vi "test_config_file_generator.vi"() -> ()   [LabVIEW 2019]
uses:
  RT/RT Controls/Main Box Config.ctl
  <vilib>/Utility/config.llb/Config Data RefNum.ctl
  <vilib>/Utility/config.llb/Write Key (I32).vi
  <vilib>/Utility/config.llb/Write Key (Double).vi
  <vilib>/Utility/config.llb/Write Key (Boolean).vi
  <vilib>/Utility/config.llb/Write Key (U32).vi
  <vilib>/Utility/config.llb/Read Key (I32).vi
  <vilib>/Utility/config.llb/Read Key (Double).vi
  <vilib>/Utility/config.llb/Read Key (Boolean).vi
  <vilib>/Utility/config.llb/NI_LVConfig.lvlib
panel:
  out "out":T2 {"MainBoxConfig"."Tol" format="%.2f"; "MainBoxConfig"."EncRefDeg" format="%.2f"; "MainBoxConfig"."HomePos" format="%.2f"; "MainBoxConfig"."HSThres" format="%.2f"; "MainBoxConfig"."Coast" format="%.2f"}
  in  "AzEncNoError":u16=1025
  out "error out":errorcluster
  out "key names":string[](array[string])
  out "section exists?":bool
  out "file refnum":T3
  in  "MainHostTO":u16=60
  in  "MainHostPort":u16=17310
  in  "TopUDPPort":u16=17308
  in  "config path":path=path "C:/Users/norman/Documents/test/soar_dome/test/config.ini"
  in  "MainBoxConfig":T1={"WatchdogTim"=600, "DirRevDel"=4, "Coast"=0.5, "HSThres"=5.0, "EncCounts360"=4018143232, "HomePos"=0.0, "EncRefDeg"=0.0, "EncRefCounts"=79895940197, "Tol"=1.0, "CloudEn"=FALSE, "AutoShutEn"=FALSE, "RainTim"=5, "AZTimeout"=120, "AZEncPol"=enum."Positive"} caption="value" {"Tol" format="%.2f"; "EncRefDeg" format="%.2f"; "HomePos" format="%.2f"; "HSThres" format="%.2f"; "Coast" format="%.2f"}
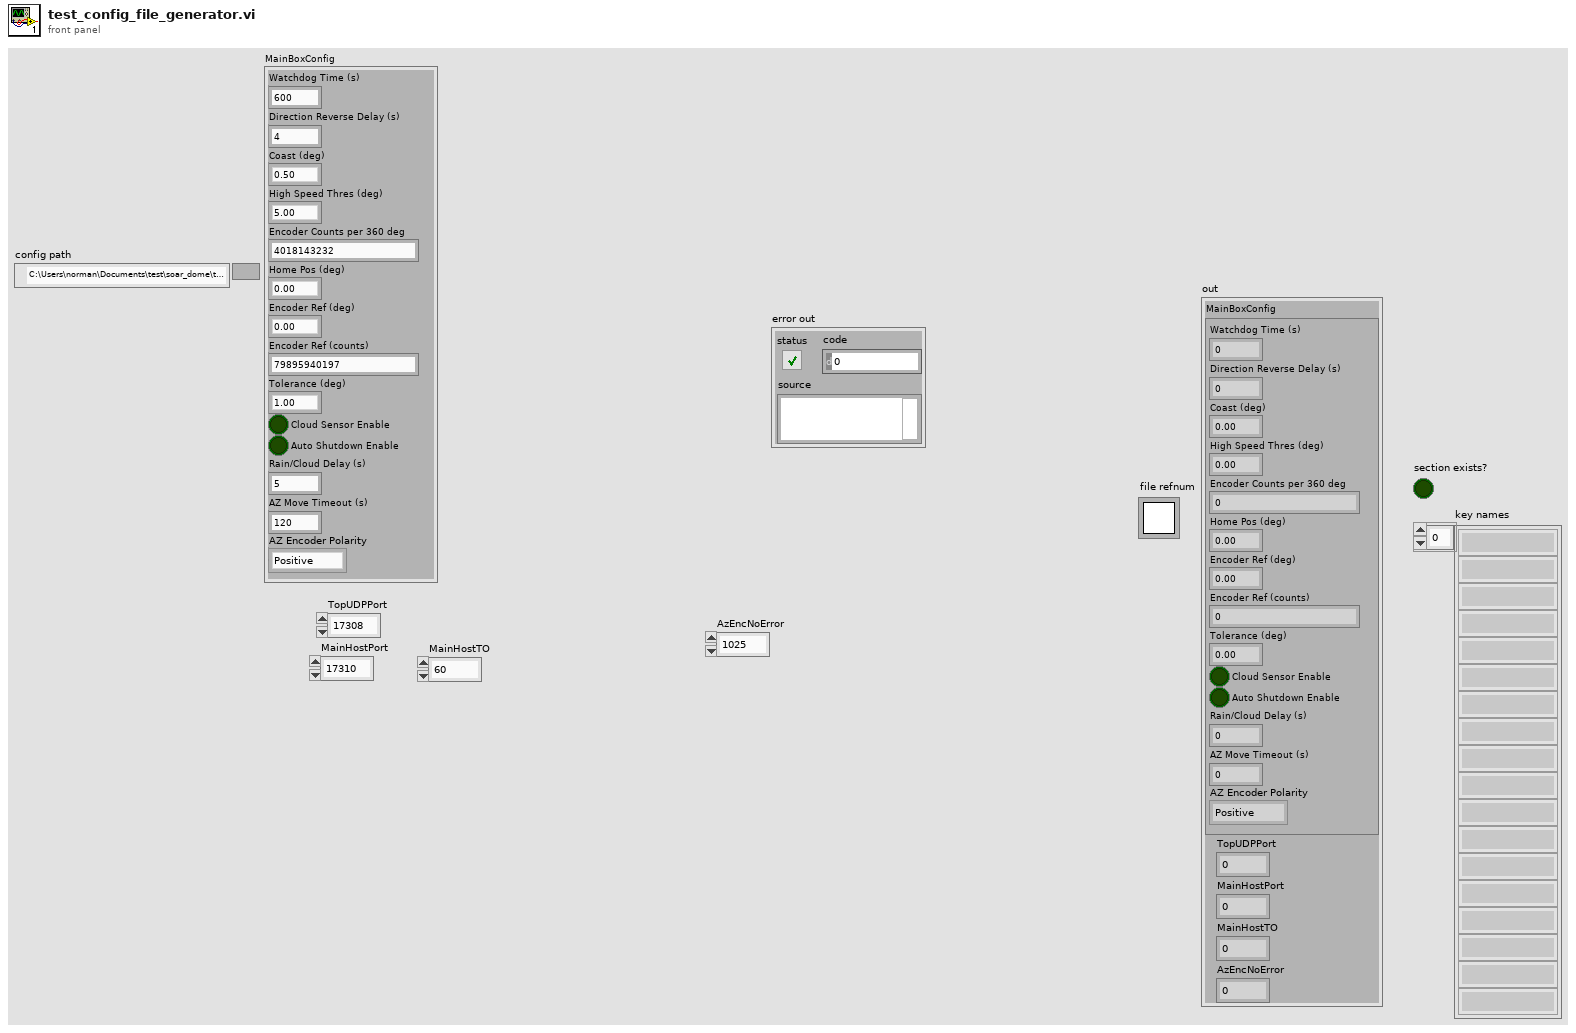
[diagram p1: front panel]
types:
  T1 = typedef "Main Box Config.ctl" = cluster{"WatchdogTim":i32, "DirRevDel":i32, "Coast":dbl, "HSThres":dbl, "EncCounts360":u64, "HomePos":dbl, "EncRefDeg":dbl, "EncRefCounts":u64, "Tol":dbl, "CloudEn":bool, "AutoShutEn":bool, "RainTim":i32, "AZTimeout":i32, "AZEncPol":enum16{"Positive", "Negative"}}
  T2 = cluster{"MainBoxConfig":T1, "TopUDPPort":u16, "MainHostPort":u16, "MainHostTO":u16, "AzEncNoError":u16}
  T3 = typedef "NI_LVConfig.lvlib/Config Data RefNum.ctl" = refnum<k1>
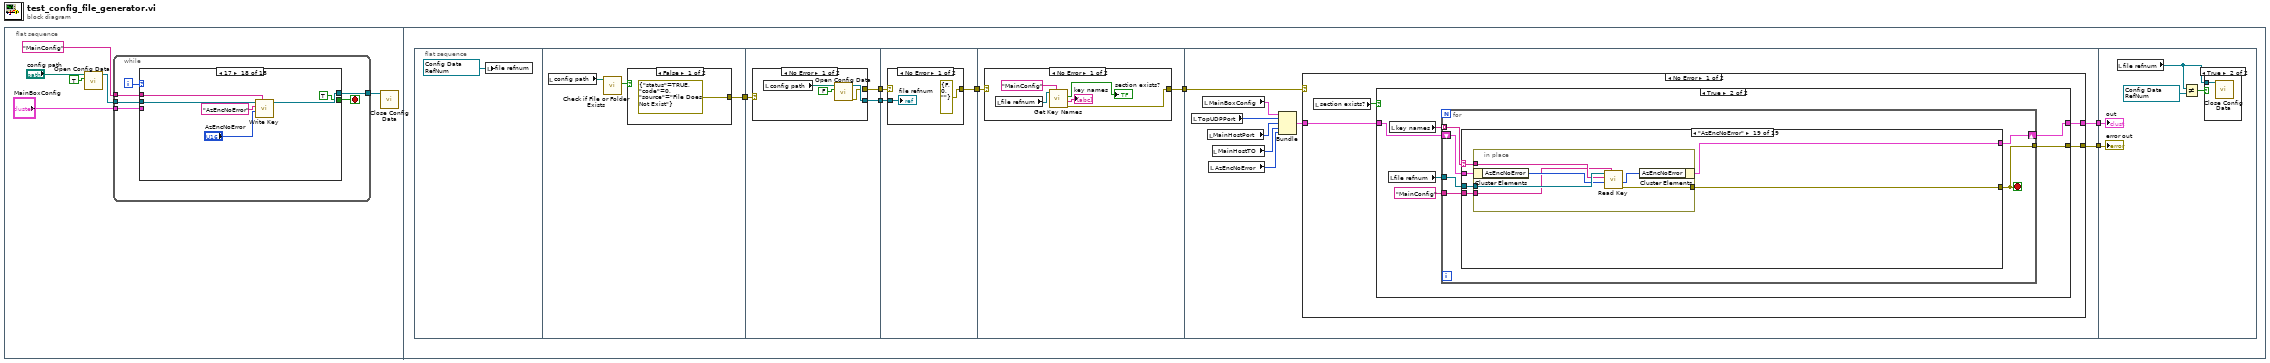
[diagram p0: block diagram]
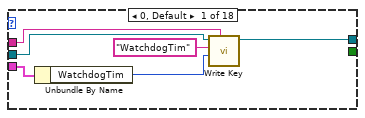
[diagram p2: hidden frame]
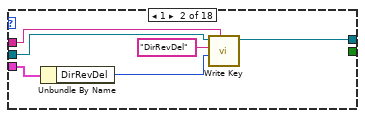
[diagram p3: hidden frame]
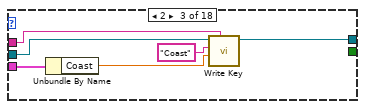
[diagram p4: hidden frame]
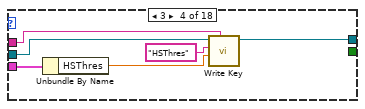
[diagram p5: hidden frame]
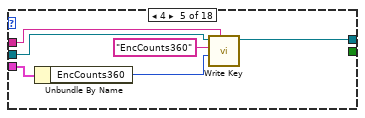
[diagram p6: hidden frame]
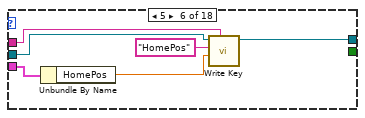
[diagram p7: hidden frame]
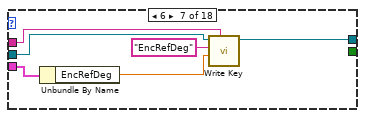
[diagram p8: hidden frame]
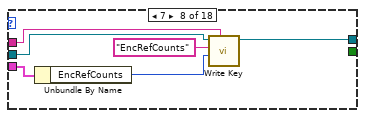
[diagram p9: hidden frame]
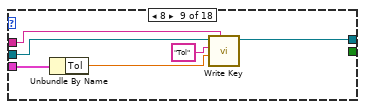
[diagram p10: hidden frame]
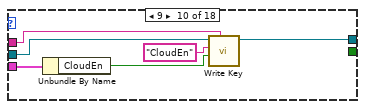
[diagram p11: hidden frame]
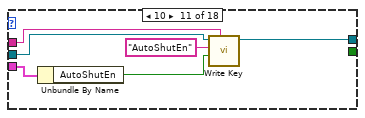
[diagram p12: hidden frame]
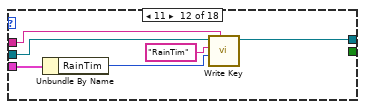
[diagram p13: hidden frame]
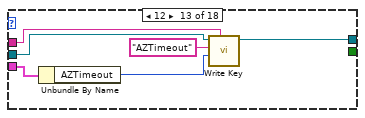
[diagram p14: hidden frame]
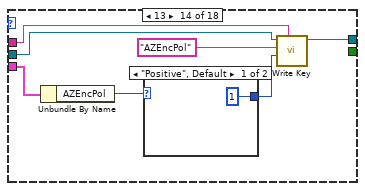
[diagram p15: hidden frame]
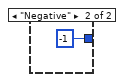
[diagram p16: hidden frame]
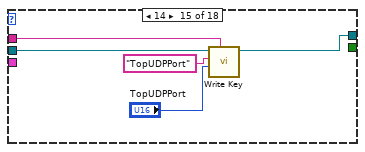
[diagram p17: hidden frame]
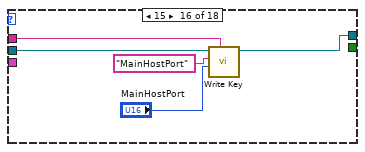
[diagram p18: hidden frame]
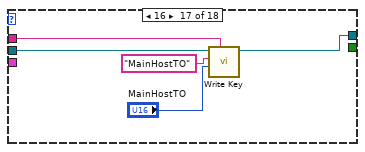
[diagram p19: hidden frame]
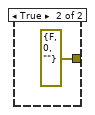
[diagram p20: hidden frame]
diagram:
  n1 = flat-sequence {
    frame #0 {
      n2 = call <vilib>:"Open Config Data.vi"("create file if necessary (T)"=TRUE, "configuration file path"="config path") -> ("refnum"=w4:T3)  [unwired: 7 in, 2 out]
      n3 = while {
        tunnel: w4 -> [w10]
        tunnel: "MainConfig" ("section") -> [w11]
        tunnel: [w9] -> w1
        tunnel: "MainBoxConfig" -> [w8]
        i -> [w12]
        stop <- w7 stop-if-true
        n4 = case shown="17" w12 {
          tunnel: w11 -> [w18 w24 w30 w36 w42 w48 w54 w60 w66 w72 w78 w84 w90 w97 w103 w108 w113 w119]
          tunnel: w10 -> [w17 w23 w29 w35 w41 w47 w53 w59 w65 w71 w77 w83 w89 w96 w104 w109 w114 w120]
          tunnel: [w16 w22 w28 w34 w40 w46 w52 w58 w64 w70 w76 w82 w88 w95 w100 w106 w111 w117] -> w9
          tunnel: w8 -> [w14 w20 w26 w32 w38 w44 w50 w56 w62 w68 w74 w80 w86 w93 _ _ _ _]
          tunnel: [_ _ _ _ _ _ _ _ _ _ _ _ _ _ _ _ _ TRUE] -> w7
          frame 0, Default {
            n5 = Unbundle By Name(w14) -> ("WatchdogTim"=w13:i32)
            n6 = call-poly <vilib>:"Write Key.vi"("section"=w18, "value"=w13, "key"="WatchdogTim", "refnum"=w17) -> ("refnum out"=w16:T3)  [unwired: 5 in, 2 out]
          }
          frame 1 {
            n7 = Unbundle By Name(w20) -> ("DirRevDel"=w19:i32)
            n8 = call-poly <vilib>:"Write Key.vi"("section"=w24, "value"=w19, "key"="DirRevDel", "refnum"=w23) -> ("refnum out"=w22:T3)  [unwired: 5 in, 2 out]
          }
          frame 2 {
            n9 = Unbundle By Name(w26) -> ("Coast"=w25:dbl)
            n10 = call-poly <vilib>:"Write Key.vi"("section"=w30, "value"=w25, "key"="Coast", "refnum"=w29) -> ("refnum out"=w28:T3)  [unwired: 5 in, 2 out]
          }
          frame 3 {
            n11 = Unbundle By Name(w32) -> ("HSThres"=w31:dbl)
            n12 = call-poly <vilib>:"Write Key.vi"("section"=w36, "value"=w31, "key"="HSThres", "refnum"=w35) -> ("refnum out"=w34:T3)  [unwired: 5 in, 2 out]
          }
          frame 4 {
            n13 = Unbundle By Name(w38) -> ("EncCounts360"=w37:u64)
            n14 = call-poly <vilib>:"Write Key.vi"("section"=w42, "value"=w37, "key"="EncCounts360", "refnum"=w41) -> ("refnum out"=w40:T3)  [unwired: 5 in, 2 out]
          }
          frame 5 {
            n15 = Unbundle By Name(w44) -> ("HomePos"=w43:dbl)
            n16 = call-poly <vilib>:"Write Key.vi"("section"=w48, "value"=w43, "key"="HomePos", "refnum"=w47) -> ("refnum out"=w46:T3)  [unwired: 5 in, 2 out]
          }
          frame 6 {
            n17 = Unbundle By Name(w50) -> ("EncRefDeg"=w49:dbl)
            n18 = call-poly <vilib>:"Write Key.vi"("section"=w54, "value"=w49, "key"="EncRefDeg", "refnum"=w53) -> ("refnum out"=w52:T3)  [unwired: 5 in, 2 out]
          }
          frame 7 {
            n19 = Unbundle By Name(w56) -> ("EncRefCounts"=w55:u64)
            n20 = call-poly <vilib>:"Write Key.vi"("section"=w60, "value"=w55, "key"="EncRefCounts", "refnum"=w59) -> ("refnum out"=w58:T3)  [unwired: 5 in, 2 out]
          }
          frame 8 {
            n21 = Unbundle By Name(w62) -> ("Tol"=w61:dbl)
            n22 = call-poly <vilib>:"Write Key.vi"("section"=w66, "value"=w61, "key"="Tol", "refnum"=w65) -> ("refnum out"=w64:T3)  [unwired: 5 in, 2 out]
          }
          frame 9 {
            n23 = Unbundle By Name(w68) -> ("CloudEn"=w67:bool)
            n24 = call-poly <vilib>:"Write Key.vi"("section"=w72, "value"=w67, "key"="CloudEn", "refnum"=w71) -> ("refnum out"=w70:T3)  [unwired: 5 in, 2 out]
          }
          frame 10 {
            n25 = Unbundle By Name(w74) -> ("AutoShutEn"=w73:bool)
            n26 = call-poly <vilib>:"Write Key.vi"("section"=w78, "value"=w73, "key"="AutoShutEn", "refnum"=w77) -> ("refnum out"=w76:T3)  [unwired: 5 in, 2 out]
          }
          frame 11 {
            n27 = Unbundle By Name(w80) -> ("RainTim"=w79:i32)
            n28 = call-poly <vilib>:"Write Key.vi"("section"=w84, "value"=w79, "key"="RainTim", "refnum"=w83) -> ("refnum out"=w82:T3)  [unwired: 5 in, 2 out]
          }
          frame 12 {
            n29 = Unbundle By Name(w86) -> ("AZTimeout"=w85:i32)
            n30 = call-poly <vilib>:"Write Key.vi"("section"=w90, "value"=w85, "key"="AZTimeout", "refnum"=w89) -> ("refnum out"=w88:T3)  [unwired: 5 in, 2 out]
          }
          frame 13 {
            n31 = Unbundle By Name(w93) -> ("AZEncPol"=w92:enum16{"Positive", "Negative"})
            n32 = case shown="\"Positive\", Default" w92 {
              tunnel: [1 -1] -> w91
              frame "Positive", Default {
              }
              frame "Negative" {
              }
            }
            n33 = call-poly <vilib>:"Write Key.vi"("section"=w97, "value"=w91, "key"="AZEncPol", "refnum"=w96) -> ("refnum out"=w95:T3)  [unwired: 5 in, 2 out]
          }
          frame 14 {
            n34 = call-poly <vilib>:"Write Key.vi"("section"=w103, "value"="TopUDPPort", "key"="TopUDPPort", "refnum"=w104) -> ("refnum out"=w100:T3)  [unwired: 5 in, 2 out]
          }
          frame 15 {
            n35 = call-poly <vilib>:"Write Key.vi"("section"=w108, "value"="MainHostPort", "key"="MainHostPort", "refnum"=w109) -> ("refnum out"=w106:T3)  [unwired: 5 in, 2 out]
          }
          frame 16 {
            n36 = call-poly <vilib>:"Write Key.vi"("section"=w113, "value"="MainHostTO", "key"="MainHostTO", "refnum"=w114) -> ("refnum out"=w111:T3)  [unwired: 5 in, 2 out]
          }
          frame 17 {
            n37 = call-poly <vilib>:"Write Key.vi"("section"=w119, "value"="AzEncNoError", "key"="AzEncNoError", "refnum"=w120) -> ("refnum out"=w117:T3)  [unwired: 5 in, 2 out]
          }
        }
      }
      n38 = call <vilib>:"Close Config Data.vi"("refnum"=w1) -> ()  [unwired: 9 in, 2 out]
    }
    frame #1 {
      n39 = flat-sequence {
        tunnel: [w129] -> w127
        tunnel: w127 -> [w136]
        tunnel: [w135] -> w126
        tunnel: [w134] -> w125
        tunnel: w126 -> [w144]
        tunnel: w125 -> [w145]
        tunnel: [w143] -> w124
        tunnel: w124 -> [w150]
        tunnel: [w149] -> w123
        tunnel: w123 -> [w160]
        tunnel: [w159] -> w122
        tunnel: [w158] -> w121
        tunnel: w122 -> [w414]
        tunnel: w121 -> [w410]
        frame #0 {
          w128 = T3 refnum items=["config data"] ("file refnum")
          n40 = local write "file refnum"(w128) -> ()
        }
        frame #1 {
          n41 = local read "config path"() -> (w130:path)
          n42 = call <vilib>:"Check if File or Folder Exists.vi"("path"=w130) -> ("file or folder exists?"=w131:bool)  [unwired: 8 in, 2 out]
          n43 = case shown="False" w131 {
            tunnel: [errorcluster {"status"=TRUE, "code"=0, "source"="File Does Not Exist"} ("error constant") errorcluster {"status"=FALSE, "code"=0, "source"=""} ("error constant")] -> w129
            frame False {
            }
            frame True {
            }
          }
        }
        frame #2 {
          n44 = case shown="No Error" w136 {
            selector: w136 -> [_ w141]
            tunnel: [w139 w142] -> w135
            tunnel: [w138 w141] -> w134
            frame No Error {
              n45 = local read "config path"() -> (w140:path)
              n46 = call <vilib>:"Open Config Data.vi"("create file if necessary (T)"=FALSE, "configuration file path"=w140) -> ("error out"=w138:errorcluster, "refnum"=w139:T3)  [unwired: 7 in, 1 out]
            }
            frame Error {
              w142 = T3 refnum items=["config data"] ("refnum")
            }
          }
        }
        frame #3 {
          n47 = case shown="No Error" w145 {
            selector: w145 -> [_ w148]
            tunnel: w144 -> [w147 _]
            tunnel: [errorcluster {"status"=FALSE, "code"=0, "source"=""} ("error IO") w148] -> w143
            frame No Error {
              "file refnum" <- w147
            }
            frame Error {
            }
          }
        }
        frame #4 {
          n48 = case shown="No Error" w150 {
            selector: w150 -> [_ w156]
            tunnel: [w153 w156] -> w149
            frame No Error {
              n49 = local read "file refnum"() -> (w155:T3)
              n50 = call <vilib>:"Get Key Names.vi"("section"="MainConfig", "refnum"=w155) -> ("error out"=w153:errorcluster, "key names"=→"key names":string[], "section exists?"=→"section exists?":bool)  [unwired: 6 in, 1 out]
            }
            frame Error {
            }
          }
        }
        frame #5 {
          n51 = local read "TopUDPPort"() -> (w163:u16)
          n52 = local read "MainBoxConfig"() -> (w164:T1)
          n53 = local read "MainHostPort"() -> (w162:u16)
          n54 = local read "AzEncNoError"() -> (w157:u16)
          n55 = local read "MainHostTO"() -> (w161:u16)
          n56 = Bundle("MainBoxConfig"=w164, "TopUDPPort"=w163, "MainHostPort"=w162, "MainHostTO"=w161, "AzEncNoError"=w157) -> (w165:T2)  [unwired: 1 in]
          n57 = case shown="No Error" w160 {
            selector: w160 -> [_ w408]
            tunnel: [w169 w409] -> w158
            tunnel: w165 -> [w168 w409]
            tunnel: [w166 w408] -> w159
            frame No Error {
              n58 = local read "section exists?"() -> (w167:bool)
              n59 = case shown="True" w167 {
                tunnel: w168 -> [w171 w177]
                tunnel: [w171 w176] -> w169
                tunnel: [errorcluster {"status"=FALSE, "code"=0, "source"=""} ("error out") w175] -> w166
                frame False {
                }
                frame True {
                  n60 = local read "file refnum"() -> (w172:T3)
                  n61 = local read "key names"() -> (w174:string[])
                  n62 = for {
                    tunnel: w174 -> [w183] mode=indexing
                    tunnel: w172 -> [w182]
                    shift-right: [w180] -> w176
                    shift-left: w177 -> [w181]
                    tunnel: "MainConfig" ("section") -> [w179]
                    tunnel: [w178] -> w175
                    stop <- w178 stop-if-true
                    n63 = case shown="\"AzEncNoError\"" w183 {
                      selector: w183 -> [_ w188 w200 w212 w224 w235 w247 w259 w271 w283 w295 w307 w319 w331 w343 w361 w373 w385 w397]
                      tunnel: w182 -> [_ w189 w201 w213 w225 w237 w249 w261 w273 w285 w297 w309 w321 w333 w345 w362 w374 w386 w398]
                      tunnel: w181 -> [w185 w191 w203 w215 w227 w239 w251 w263 w275 w287 w299 w311 w323 w335 w347 w365 w377 w389 w401]
                      tunnel: [w185 w190 w202 w214 w226 w238 w250 w262 w274 w286 w298 w310 w322 w334 w346 w364 w376 w388 w400] -> w180
                      tunnel: w179 -> [_ w187 w199 w211 w223 w236 w248 w260 w272 w284 w296 w308 w320 w332 w344 w363 w375 w387 w399]
                      tunnel: [errorcluster {"status"=FALSE, "code"=0, "source"=""} ("error out") w186 w198 w210 w222 w234 w246 w258 w270 w282 w294 w306 w318 w330 w342 w360 w372 w384 w396] -> w178
                      frame "False", Default {
                      }
                      frame "WatchdogTim" {
                        n64 = in-place {
                          in-place-border: w189 -> [w197]
                          in-place-border: w188 -> [w194]
                          in-place-border: w187 -> [w193]
                          in-place-border: [w192] -> w186
                          n65 = in-place-cluster #1(w191) -> ("MainBoxConfig.WatchdogTim"=w196:i32)
                          n66 = call-poly <vilib>:"Read Key.vi"("section"=w193, "default value"=w196, "key"=w194, "refnum"=w197) -> ("error out"=w192:errorcluster, "value"=w195:i32)  [unwired: 4 in, 2 out]
                          n67 = in-place-cluster #1("MainBoxConfig.WatchdogTim"=w195) -> (w190:T2)
                        }
                      }
                      frame "DirRevDel" {
                        n68 = in-place {
                          in-place-border: w201 -> [w209]
                          in-place-border: w200 -> [w206]
                          in-place-border: w199 -> [w205]
                          in-place-border: [w204] -> w198
                          n69 = in-place-cluster #2(w203) -> ("MainBoxConfig.DirRevDel"=w208:i32)
                          n70 = call-poly <vilib>:"Read Key.vi"("section"=w205, "default value"=w208, "key"=w206, "refnum"=w209) -> ("error out"=w204:errorcluster, "value"=w207:i32)  [unwired: 4 in, 2 out]
                          n71 = in-place-cluster #2("MainBoxConfig.DirRevDel"=w207) -> (w202:T2)
                        }
                      }
                      frame "Coast" {
                        n72 = in-place {
                          in-place-border: w213 -> [w221]
                          in-place-border: w212 -> [w218]
                          in-place-border: w211 -> [w217]
                          in-place-border: [w216] -> w210
                          n73 = in-place-cluster #3(w215) -> ("MainBoxConfig.Coast"=w220:dbl)
                          n74 = call-poly <vilib>:"Read Key.vi"("section"=w217, "default value"=w220, "key"=w218, "refnum"=w221) -> ("error out"=w216:errorcluster, "value"=w219:dbl)  [unwired: 4 in, 2 out]
                          n75 = in-place-cluster #3("MainBoxConfig.Coast"=w219) -> (w214:T2)
                        }
                      }
                      frame "HSThres" {
                        n76 = in-place {
                          in-place-border: w225 -> [w233]
                          in-place-border: w224 -> [w230]
                          in-place-border: w223 -> [w229]
                          in-place-border: [w228] -> w222
                          n77 = in-place-cluster #4(w227) -> ("MainBoxConfig.HSThres"=w232:dbl)
                          n78 = call-poly <vilib>:"Read Key.vi"("section"=w229, "default value"=w232, "key"=w230, "refnum"=w233) -> ("error out"=w228:errorcluster, "value"=w231:dbl)  [unwired: 4 in, 2 out]
                          n79 = in-place-cluster #4("MainBoxConfig.HSThres"=w231) -> (w226:T2)
                        }
                      }
                      frame "EncCounts360" {
                        n80 = in-place {
                          in-place-border: w237 -> [w245]
                          in-place-border: w236 -> [w242]
                          in-place-border: w235 -> [w241]
                          in-place-border: [w240] -> w234
                          n81 = in-place-cluster #5(w239) -> ("MainBoxConfig.EncCounts360"=w244:u64)
                          n82 = call-poly <vilib>:"Read Key.vi"("section"=w242, "default value"=w244, "key"=w241, "refnum"=w245) -> ("error out"=w240:errorcluster, "value"=w243:dbl)  [unwired: 4 in, 2 out]
                          n83 = in-place-cluster #5("MainBoxConfig.EncCounts360"=w243) -> (w238:T2)
                        }
                      }
                      frame "HomePos" {
                        n84 = in-place {
                          in-place-border: w249 -> [w257]
                          in-place-border: w248 -> [w254]
                          in-place-border: w247 -> [w253]
                          in-place-border: [w252] -> w246
                          n85 = in-place-cluster #6(w251) -> ("MainBoxConfig.HomePos"=w256:dbl)
                          n86 = call-poly <vilib>:"Read Key.vi"("section"=w254, "default value"=w256, "key"=w253, "refnum"=w257) -> ("error out"=w252:errorcluster, "value"=w255:dbl)  [unwired: 4 in, 2 out]
                          n87 = in-place-cluster #6("MainBoxConfig.HomePos"=w255) -> (w250:T2)
                        }
                      }
                      frame "EncRefDeg" {
                        n88 = in-place {
                          in-place-border: w261 -> [w269]
                          in-place-border: w260 -> [w266]
                          in-place-border: w259 -> [w265]
                          in-place-border: [w264] -> w258
                          n89 = in-place-cluster #7(w263) -> ("MainBoxConfig.EncRefDeg"=w268:dbl)
                          n90 = call-poly <vilib>:"Read Key.vi"("section"=w266, "default value"=w268, "key"=w265, "refnum"=w269) -> ("error out"=w264:errorcluster, "value"=w267:dbl)  [unwired: 4 in, 2 out]
                          n91 = in-place-cluster #7("MainBoxConfig.EncRefDeg"=w267) -> (w262:T2)
                        }
                      }
                      frame "EncRefCounts" {
                        n92 = in-place {
                          in-place-border: w273 -> [w281]
                          in-place-border: w272 -> [w278]
                          in-place-border: w271 -> [w277]
                          in-place-border: [w276] -> w270
                          n93 = in-place-cluster #8(w275) -> ("MainBoxConfig.EncRefCounts"=w280:u64)
                          n94 = call-poly <vilib>:"Read Key.vi"("section"=w278, "default value"=w280, "key"=w277, "refnum"=w281) -> ("error out"=w276:errorcluster, "value"=w279:dbl)  [unwired: 4 in, 2 out]
                          n95 = in-place-cluster #8("MainBoxConfig.EncRefCounts"=w279) -> (w274:T2)
                        }
                      }
                      frame "Tol" {
                        n96 = in-place {
                          in-place-border: w285 -> [w293]
                          in-place-border: w284 -> [w290]
                          in-place-border: w283 -> [w289]
                          in-place-border: [w288] -> w282
                          n97 = in-place-cluster #9(w287) -> ("MainBoxConfig.Tol"=w292:dbl)
                          n98 = call-poly <vilib>:"Read Key.vi"("section"=w290, "default value"=w292, "key"=w289, "refnum"=w293) -> ("error out"=w288:errorcluster, "value"=w291:dbl)  [unwired: 4 in, 2 out]
                          n99 = in-place-cluster #9("MainBoxConfig.Tol"=w291) -> (w286:T2)
                        }
                      }
                      frame "CloudEn" {
                        n100 = in-place {
                          in-place-border: w297 -> [w305]
                          in-place-border: w296 -> [w302]
                          in-place-border: w295 -> [w301]
                          in-place-border: [w300] -> w294
                          n101 = in-place-cluster #10(w299) -> ("MainBoxConfig.CloudEn"=w304:bool)
                          n102 = call-poly <vilib>:"Read Key.vi"("section"=w302, "default value"=w304, "key"=w301, "refnum"=w305) -> ("error out"=w300:errorcluster, "value"=w303:bool)  [unwired: 4 in, 2 out]
                          n103 = in-place-cluster #10("MainBoxConfig.CloudEn"=w303) -> (w298:T2)
                        }
                      }
                      frame "AutoShutEn" {
                        n104 = in-place {
                          in-place-border: w309 -> [w317]
                          in-place-border: w308 -> [w314]
                          in-place-border: w307 -> [w313]
                          in-place-border: [w312] -> w306
                          n105 = in-place-cluster #11(w311) -> ("MainBoxConfig.AutoShutEn"=w316:bool)
                          n106 = call-poly <vilib>:"Read Key.vi"("section"=w314, "default value"=w316, "key"=w313, "refnum"=w317) -> ("error out"=w312:errorcluster, "value"=w315:bool)  [unwired: 4 in, 2 out]
                          n107 = in-place-cluster #11("MainBoxConfig.AutoShutEn"=w315) -> (w310:T2)
                        }
                      }
                      frame "RainTim" {
                        n108 = in-place {
                          in-place-border: w321 -> [w329]
                          in-place-border: w320 -> [w326]
                          in-place-border: w319 -> [w325]
                          in-place-border: [w324] -> w318
                          n109 = in-place-cluster #12(w323) -> ("MainBoxConfig.RainTim"=w328:i32)
                          n110 = call-poly <vilib>:"Read Key.vi"("section"=w326, "default value"=w328, "key"=w325, "refnum"=w329) -> ("error out"=w324:errorcluster, "value"=w327:i32)  [unwired: 4 in, 2 out]
                          n111 = in-place-cluster #12("MainBoxConfig.RainTim"=w327) -> (w322:T2)
                        }
                      }
                      frame "AZTimeout" {
                        n112 = in-place {
                          in-place-border: w333 -> [w341]
                          in-place-border: w332 -> [w338]
                          in-place-border: w331 -> [w337]
                          in-place-border: [w336] -> w330
                          n113 = in-place-cluster #13(w335) -> ("MainBoxConfig.AZTimeout"=w340:i32)
                          n114 = call-poly <vilib>:"Read Key.vi"("section"=w338, "default value"=w340, "key"=w337, "refnum"=w341) -> ("error out"=w336:errorcluster, "value"=w339:i32)  [unwired: 4 in, 2 out]
                          n115 = in-place-cluster #13("MainBoxConfig.AZTimeout"=w339) -> (w334:T2)
                        }
                      }
                      frame "AZEncPol" {
                        n116 = in-place {
                          in-place-border: w345 -> [w355]
                          in-place-border: w344 -> [w354]
                          in-place-border: w343 -> [w353]
                          in-place-border: [w348] -> w342
                          n117 = in-place-cluster #14(w347) -> ("MainBoxConfig.AZEncPol"=w352:enum16{"Positive", "Negative"})
                          n118 = case shown="\"Positive\", Default" w352 {
                            tunnel: [1 -1] -> w351
                            frame "Positive", Default {
                            }
                            frame "Negative" {
                            }
                          }
                          n119 = call-poly <vilib>:"Read Key.vi"("section"=w354, "default value"=w351, "key"=w353, "refnum"=w355) -> ("error out"=w348:errorcluster, "value"=w350:i32)  [unwired: 4 in, 2 out]
                          n120 = case shown="1, Default" w350 {
                            tunnel: [enum16{"Positive", "Negative"}."Negative" ("AZEncPol") enum16{"Positive", "Negative"}."Positive" ("AZEncPol")] -> w349
                            frame -1 {
                            }
                            frame 1, Default {
                            }
                          }
                          n121 = in-place-cluster #14("MainBoxConfig.AZEncPol"=w349) -> (w346:T2)
                        }
                      }
                      frame "TopUDPPort" {
                        n122 = in-place {
                          in-place-border: w362 -> [w371]
                          in-place-border: w361 -> [w368]
                          in-place-border: w363 -> [w367]
                          in-place-border: [w366] -> w360
                          n123 = in-place-cluster #15(w365) -> ("TopUDPPort"=w370:u16)
                          n124 = call-poly <vilib>:"Read Key.vi"("section"=w367, "default value"=w370, "key"=w368, "refnum"=w371) -> ("error out"=w366:errorcluster, "value"=w369:i32)  [unwired: 4 in, 2 out]
                          n125 = in-place-cluster #15("TopUDPPort"=w369) -> (w364:T2)
                        }
                      }
                      frame "MainHostPort" {
                        n126 = in-place {
                          in-place-border: w374 -> [w383]
                          in-place-border: w373 -> [w380]
                          in-place-border: w375 -> [w379]
                          in-place-border: [w378] -> w372
                          n127 = in-place-cluster #16(w377) -> ("MainHostPort"=w382:u16)
                          n128 = call-poly <vilib>:"Read Key.vi"("section"=w379, "default value"=w382, "key"=w380, "refnum"=w383) -> ("error out"=w378:errorcluster, "value"=w381:i32)  [unwired: 4 in, 2 out]
                          n129 = in-place-cluster #16("MainHostPort"=w381) -> (w376:T2)
                        }
                      }
                      frame "MainHostTO" {
                        n130 = in-place {
                          in-place-border: w386 -> [w395]
                          in-place-border: w385 -> [w392]
                          in-place-border: w387 -> [w391]
                          in-place-border: [w390] -> w384
                          n131 = in-place-cluster #17(w389) -> ("MainHostTO"=w394:u16)
                          n132 = call-poly <vilib>:"Read Key.vi"("section"=w391, "default value"=w394, "key"=w392, "refnum"=w395) -> ("error out"=w390:errorcluster, "value"=w393:i32)  [unwired: 4 in, 2 out]
                          n133 = in-place-cluster #17("MainHostTO"=w393) -> (w388:T2)
                        }
                      }
                      frame "AzEncNoError" {
                        n134 = in-place {
                          in-place-border: w398 -> [w407]
                          in-place-border: w397 -> [w404]
                          in-place-border: w399 -> [w403]
                          in-place-border: [w402] -> w396
                          n135 = in-place-cluster #18(w401) -> ("AzEncNoError"=w406:u16)
                          n136 = call-poly <vilib>:"Read Key.vi"("section"=w403, "default value"=w406, "key"=w404, "refnum"=w407) -> ("error out"=w402:errorcluster, "value"=w405:i32)  [unwired: 4 in, 2 out]
                          n137 = in-place-cluster #18("AzEncNoError"=w405) -> (w400:T2)
                        }
                      }
                    }
                  }
                }
              }
            }
            frame Error {
            }
          }
        }
        frame #6 {
          w411 = T3 refnum items=["config data"] ("y")
          n138 = local read "file refnum"() -> (w413:T3)
          n139 = Not Equal?(x=w413, y=w411) -> (x != y?=w412:bool)
          n140 = case shown="True" w412 {
            tunnel: w413 -> [_ w415]
            frame False {
            }
            frame True {
              n141 = call <vilib>:"Close Config Data.vi"("refnum"=w415) -> ()  [unwired: 9 in, 2 out]
            }
          }
          "error out" <- w414
          "out" <- w410
        }
      }
    }
  }
